vi "DiffCondSRS830.vi"() -> ()   [LabVIEW 2020]
panel:
  out "XY Graph":cluster{dbl[], dbl[]}(graph)
  out "Resistance":dbl[](array[numeric])
  out "Current":dbl[](array[numeric])
  out "Voltage":dbl[](array[numeric])
  in  "Keithley 2182A Address":refnum<visa-resource-name>
  in  "SRS 830 Address":refnum<visa-resource-name>
  in  "Delay (S)":dbl=0.3
  in  "Freq (Hz)":dbl=314.1
  in  "Max Offset (nA)":dbl=50.0
  in  "#Steps":i32=100
  in  "Amplitude (nA)":dbl=2.5
  in  "Keithley 6221 Address":refnum<visa-resource-name>
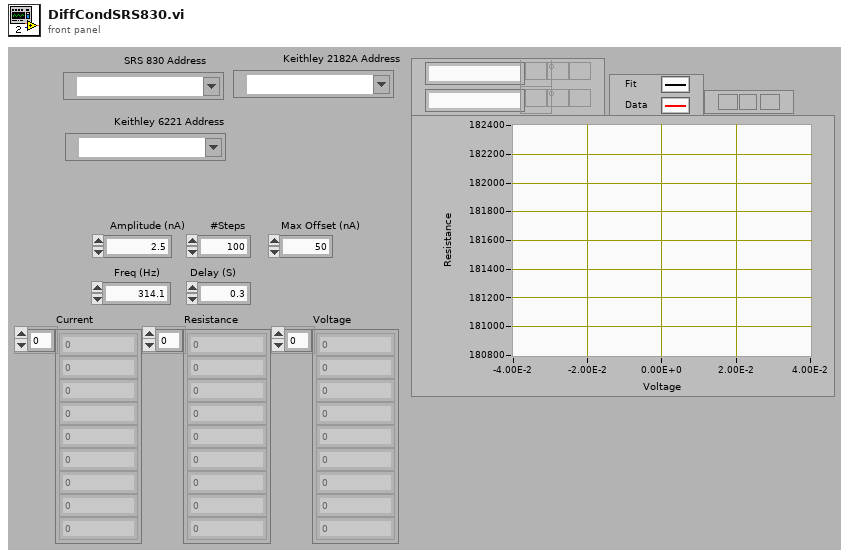
[diagram p1: front panel]
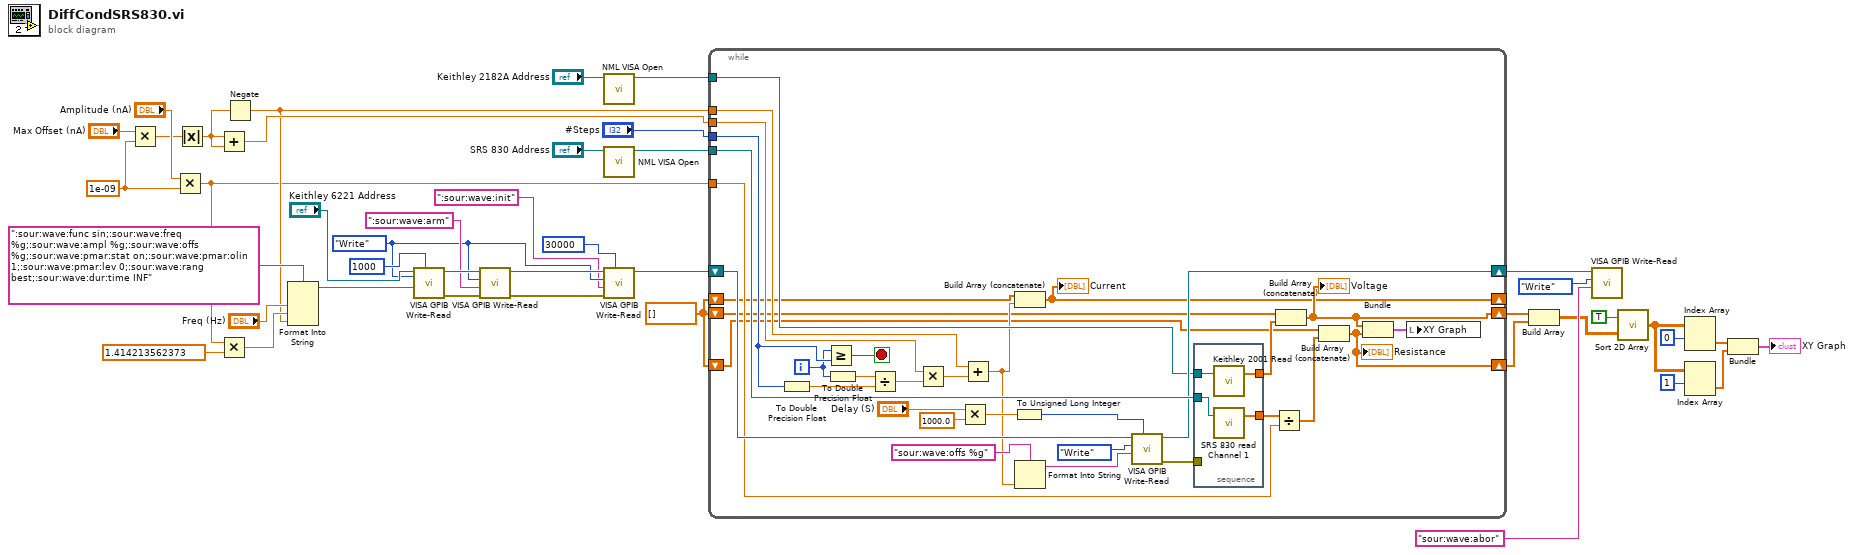
[diagram p0: block diagram]
diagram:
  w14 = dbl[] []
  w29 = enum16{"Write", "Read", "Write & Read"}."Write" ("Action")
  w19 = 1e-09 ("y")
  n1 = Multiply(x="Max Offset (nA)", y=w19) -> (x*y=w18:dbl)
  n2 = Multiply(x="Amplitude (nA)", y=w19) -> (x*y=w3:dbl)
  n3 = Absolute Value(x=w18) -> (abs(x)=w16:dbl)
  n4 = Add(x=w16, y=w16) -> (x+y=w34:dbl)
  n5 = Multiply(x=w3, y=1.414213562373) -> (x*y=w21:dbl)
  n6 = Negate(x=w16) -> (-x=w17:dbl)
  n7 = Format Into String(format string=":sour:wave:func sin;:sour:wave:freq %g;:sour:wave:ampl %g;:sour:wave:offs %g;:sour:wave:pmar:stat on;:sour:wave:pmar:olin 1;:sour:wave:pmar:lev 0;:sour:wave:rang best;:sour:wave:dur:time INF", "Freq (Hz)", w21, w17) -> (resulting string=w40:string)  [unwired: 2 in, 1 out]
  n8 = call "VISA GPIB Write-Read.vi"("Wait (ms)"=u32 1000 ("wait (mS)"), "Command"=w40, "Action"=w29, "VISA resource name"="Keithley 6221 Address") -> ("error out"=w37:errorcluster, "dup VISA Session"=w36:refnum<visa-resource-name>)  [unwired: 4 in, 2 out]
  n9 = call "VISA GPIB Write-Read.vi"("error in (no error)"=w37, "Command"=":sour:wave:arm" ("String to Write"), "Action"=w29, "VISA resource name"=w36) -> ("error out"=w32:errorcluster, "dup VISA Session"=w31:refnum<visa-resource-name>)  [unwired: 4 in, 2 out]
  n10 = call "NML VISA Open.vi"("VISA resource name"="Keithley 2182A Address") -> ("VISA resource name out"=w1:refnum<visa-resource-name>)  [unwired: 9 in, 1 out]
  n11 = call "NML VISA Open.vi"("VISA resource name"="SRS 830 Address") -> ("VISA resource name out"=w2:refnum<visa-resource-name>)  [unwired: 9 in, 1 out]
  n12 = call "VISA GPIB Write-Read.vi"("Wait (ms)"=u32 30000 ("wait (mS)"), "error in (no error)"=w32, "Command"=":sour:wave:init" ("String to Write"), "Action"=w29, "VISA resource name"=w31) -> ("dup VISA Session"=w30:refnum<visa-resource-name>)  [unwired: 3 in, 3 out]
  n13 = while {
    tunnel: "#Steps" -> [w76]
    tunnel: w17 -> [w72]
    tunnel: w34 -> [w74]
    tunnel: w2 -> [w63]
    tunnel: w3 -> [w56]
    tunnel: w1 -> [w55]
    shift-right: [w46] -> w6
    shift-left: w14 -> [w45]
    shift-right: [w49] -> _
    shift-left: w14 -> [w47]
    shift-right: [w50] -> w5
    shift-left: w14 -> [w48]
    shift-right: [w57] -> w26
    shift-left: w30 -> [w65]
    i -> [w60]
    stop <- w61 stop-if-true
    n14 = To Double Precision Float(number=w76) -> (double precision float=w58:dbl)
    n15 = Greater Or Equal?(x=w60, y=w76) -> (x >= y?=w61:bool)
    n16 = To Double Precision Float(number=w60) -> (double precision float=w59:dbl)
    n17 = Divide(x=w59, y=w58) -> (x/y=w75:dbl)
    n18 = Multiply(x=w74, y=w75) -> (x*y=w73:dbl)
    n19 = Multiply(x="Delay (S)", y=1000.0) -> (x*y=w68:dbl)
    n20 = Add(x=w72, y=w73) -> (x+y=w51:dbl)
    n21 = To Unsigned Long Integer(number=w68) -> (unsigned 32bit integer=w64:u32)
    n22 = Build Array (concatenate)(w47, w51) -> (w49:dbl[])
    "Current" <- w49
    n23 = Format Into String(format string="sour:wave:offs %g", w51) -> (resulting string=w67:string)  [unwired: 2 in, 1 out]
    n24 = call "VISA GPIB Write-Read.vi"("Wait (ms)"=w64, "Command"=w67, "Action"=enum16{"Write", "Read", "Write & Read"}."Write", "VISA resource name"=w65) -> ("error out"=w62:errorcluster, "dup VISA Session"=w57:refnum<visa-resource-name>)  [unwired: 4 in, 2 out]
    n25 = stacked-sequence {
      tunnel: w63 -> [w80]
      tunnel: w62 -> [_]
      tunnel: [w79] -> w54
      tunnel: w55 -> [w78]
      tunnel: [w77] -> w52
      frame #0 {
        n26 = call "Keithley 2001 Read.vi"("Instrument Address"=w78) -> ("Measurement"=w77:dbl[])  [unwired: 1 in, 1 out]
        n27 = call "SRS 830 read Channel 1.vi"("Instrument Address"=w80) -> ("SRS 830 Output"=w79:dbl[])  [unwired: 1 in, 1 out]
      }
    }
    n28 = Divide(x=w54, y=w56) -> (x/y=w53:dbl[])
    n29 = Build Array (concatenate)(w48, w52) -> (w50:dbl[])
    "Voltage" <- w50
    n30 = Build Array (concatenate)(w45, w53) -> (w46:dbl[])
    "Resistance" <- w46
    n31 = Bundle(w50, w46) -> (w44:cluster{dbl[], dbl[]})  [unwired: 1 in]
    n32 = local write "XY Graph"(w44) -> ()
  }
  n33 = Build Array(w5, w6) -> (w10:dbl[][])
  n34 = call "VISA GPIB Write-Read.vi"("Command"="sour:wave:abor" ("String to Write"), "Action"=enum16{"Write", "Read", "Write & Read"}."Write", "VISA resource name"=w26) -> ()  [unwired: 5 in, 4 out]
  n35 = call "Sort 2D Array.vi"(1:w10, "First Column"=TRUE) -> (0:w11:dbl[][])
  n36 = Index Array(array=w11, index (row)=0 ("disabled index (col)")) -> (element=w13:dbl[])  [unwired: 1 in]
  n37 = Index Array(array=w11, index (row)=1) -> (element=w12:dbl[])  [unwired: 1 in]
  n38 = Bundle(w13, w12) -> (→"XY Graph":cluster{dbl[], dbl[]})  [unwired: 1 in]
